vi "Get Joystick State.vi"(8 "error in (no error)":errorcluster, 10 "Joystick State":cluster{"Buttons":T1[], "Axis":T2[]}, 11 "Joystick in":refnum<class "Joystick.lvclass">) -> (0 "error out":errorcluster, 3 "Joystick out":refnum<class "Joystick.lvclass">)   [LabVIEW 2014, in "Joystick.lvlib" / "Joystick.lvclass"]
uses:
  Joystick.lvclass
  Button State.ctl
  Axis State.ctl
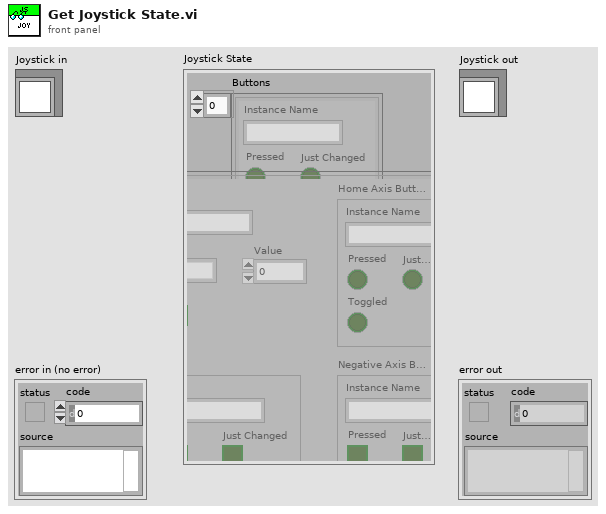
[diagram p1: front panel]
types:
  T1 = typedef "Joystick.lvlib/Joystick.lvclass/Button State.ctl" = cluster{"Pressed":bool, "Instance Name":string, "Toggled":bool, "Just Changed":bool}
  T2 = typedef "Joystick.lvlib/Joystick.lvclass/Axis State.ctl" = cluster{"Instance Name":string, "Deadband":dbl, "Value":dbl, "At Home":bool, "Postive Axis Button State":T1, "Negative Axis Button State":T1, "Home Axis Button State":T1}
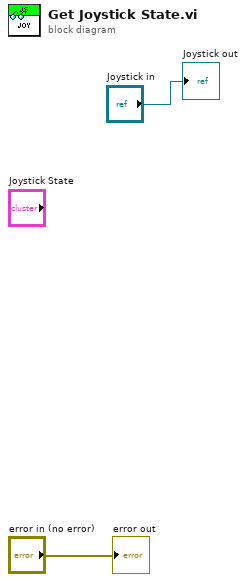
[diagram p0: block diagram]
diagram:
  "error out" <- "error in (no error)"
  "Joystick out" <- "Joystick in"
